vi "Index_Offset.vi"(10 "Offset":i32, 11 "Index":i32) -> (3 "Offset Index Out":i32)   [LabVIEW 2025]
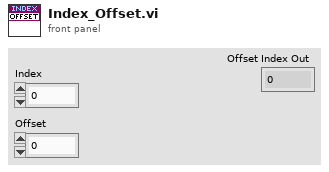
[diagram p1: front panel]
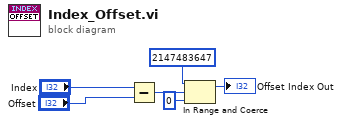
[diagram p0: block diagram]
diagram:
  n1 = Subtract(x="Index", y="Offset") -> (x-y=w4:i32)
  n2 = In Range and Coerce(upper limit=2147483647 ("32bit integer"), x=w4, lower limit=0) -> (coerced(x)=→"Offset Index Out":i32)  [unwired: 1 out]
